vi "PulseCreateDDSSeq.vi"(8 "DDS cluster IN":T2={"DDS A Cluster"={"Seq DDS freq and phase cluster"={"Seq DDS A freq cluster"={"Ch1 start /kHz"=111053.7, "Ch1 step /kHz"=0.0, "Ch2 start /kHz"=88965.3, "Ch2 step /kHz"=0.0, "Ch3 start /kHz"=113819.6, "Ch3 step /kHz"=0.0, "Ch4 start /kHz"=86210.6, "Ch4 step /kHz"=0.0}, "Seq DDS A phase cluster"={"Ch1 phase"=0.0, "Ch1 step"=0.0, "Ch2 phase"=0.0, "Ch2"=0.0, "Ch3 phase"=0.0, "Ch3 step"=0.0, "Ch4 phase"=0.0, "Ch4 step"=0.0}}, "DDS Cluster"={"freq cluster"={"C1 freq"=110584.0, "C2 freq"=111432.0, "C3 freq"=100028.0, "C4 freq"=100021.0}, "amp cluster"={"C1 amp"=0.7, "C2 amp"=0.04, "C3 amp"=0.023, "C4 amp"=0.023}, "phase cluster"={"C1 phase"=0.0, "C2 phase"=0.0, "C3 phase"=0.0, "C4 phase"=0.0}}, "Status: "=FALSE}, "DDS B Cluster"={"Seq DDS freq and phase cluster"={"Seq DDS A freq cluster"={"Ch1 start /kHz"=111053.7, "Ch1 step /kHz"=0.0, "Ch2 start /kHz"=88965.3, "Ch2 step /kHz"=0.0, "Ch3 start /kHz"=113819.6, "Ch3 step /kHz"=0.0, "Ch4 start /kHz"=86210.6, "Ch4 step /kHz"=0.0}, "Seq DDS A phase cluster"={"Ch1 phase"=0.0, "Ch1 step"=0.0, "Ch2 phase"=0.0, "Ch2"=0.0, "Ch3 phase"=0.0, "Ch3 step"=0.0, "Ch4 phase"=0.0, "Ch4 step"=0.0}}, "DDS Cluster"={"freq cluster"={"C1 freq"=110584.0, "C2 freq"=111432.0, "C3 freq"=100028.0, "C4 freq"=100021.0}, "amp cluster"={"C1 amp"=0.7, "C2 amp"=0.04, "C3 amp"=0.023, "C4 amp"=0.023}, "phase cluster"={"C1 phase"=0.0, "C2 phase"=0.0, "C3 phase"=0.0, "C4 phase"=0.0}}, "Status: "=FALSE}, "DDS C Cluster"={"Seq DDS freq and phase cluster"={"Seq DDS A freq cluster"={"Ch1 start /kHz"=111053.7, "Ch1 step /kHz"=0.0, "Ch2 start /kHz"=88965.3, "Ch2 step /kHz"=0.0, "Ch3 start /kHz"=113819.6, "Ch3 step /kHz"=0.0, "Ch4 start /kHz"=86210.6, "Ch4 step /kHz"=0.0}, "Seq DDS A phase cluster"={"Ch1 phase"=0.0, "Ch1 step"=0.0, "Ch2 phase"=0.0, "Ch2"=0.0, "Ch3 phase"=0.0, "Ch3 step"=0.0, "Ch4 phase"=0.0, "Ch4 step"=0.0}}, "DDS Cluster"={"freq cluster"={"C1 freq"=110584.0, "C2 freq"=111432.0, "C3 freq"=100028.0, "C4 freq"=100021.0}, "amp cluster"={"C1 amp"=0.7, "C2 amp"=0.04, "C3 amp"=0.023, "C4 amp"=0.023}, "phase cluster"={"C1 phase"=0.0, "C2 phase"=0.0, "C3 phase"=0.0, "C4 phase"=0.0}}, "Status: "=FALSE}, "DDS D Cluster"={"Seq DDS freq and phase cluster"={"Seq DDS A freq cluster"={"Ch1 start /kHz"=111053.7, "Ch1 step /kHz"=0.0, "Ch2 start /kHz"=88965.3, "Ch2 step /kHz"=0.0, "Ch3 start /kHz"=113819.6, "Ch3 step /kHz"=0.0, "Ch4 start /kHz"=86210.6, "Ch4 step /kHz"=0.0}, "Seq DDS A phase cluster"={"Ch1 phase"=0.0, "Ch1 step"=0.0, "Ch2 phase"=0.0, "Ch2"=0.0, "Ch3 phase"=0.0, "Ch3 step"=0.0, "Ch4 phase"=0.0, "Ch4 step"=0.0}}, "DDS Cluster"={"freq cluster"={"C1 freq"=110584.0, "C2 freq"=111432.0, "C3 freq"=100028.0, "C4 freq"=100021.0}, "amp cluster"={"C1 amp"=0.7, "C2 amp"=0.04, "C3 amp"=0.023, "C4 amp"=0.023}, "phase cluster"={"C1 phase"=0.0, "C2 phase"=0.0, "C3 phase"=0.0, "C4 phase"=0.0}}, "Status: "=FALSE}} {"DDS D Cluster"."DDS Cluster"."phase cluster"."C4 phase" min=0.0 max=0.5; "DDS D Cluster"."DDS Cluster"."phase cluster"."C3 phase" min=0.0 max=0.5; "DDS D Cluster"."DDS Cluster"."phase cluster"."C2 phase" min=0.0 max=0.5; "DDS D Cluster"."DDS Cluster"."phase cluster"."C1 phase" min=0.0 max=0.5; "DDS D Cluster"."DDS Cluster"."amp cluster"."C4 amp" min=0.0 max=0.5; "DDS D Cluster"."DDS Cluster"."amp cluster"."C3 amp" min=0.0 max=0.5; "DDS D Cluster"."DDS Cluster"."amp cluster"."C2 amp" min=0.0 max=0.5; "DDS D Cluster"."DDS Cluster"."amp cluster"."C1 amp" min=0.0 max=0.5; "DDS D Cluster"."Seq DDS freq and phase cluster"."Seq DDS A phase cluster"."Ch4 phase" format="%#_8g"; "DDS D Cluster"."Seq DDS freq and phase cluster"."Seq DDS A phase cluster"."Ch3 phase" format="%#_8g"; "DDS D Cluster"."Seq DDS freq and phase cluster"."Seq DDS A phase cluster"."Ch2 phase" format="%#_8g"; "DDS D Cluster"."Seq DDS freq and phase cluster"."Seq DDS A phase cluster"."Ch1 phase" format="%#_8g"; "DDS D Cluster"."Seq DDS freq and phase cluster"."Seq DDS A freq cluster"."Ch4 start /kHz" format="%#_8g"; "DDS D Cluster"."Seq DDS freq and phase cluster"."Seq DDS A freq cluster"."Ch3 start /kHz" format="%#_8g"; "DDS D Cluster"."Seq DDS freq and phase cluster"."Seq DDS A freq cluster"."Ch2 start /kHz" format="%#_8g"; "DDS D Cluster"."Seq DDS freq and phase cluster"."Seq DDS A freq cluster"."Ch1 start /kHz" format="%#_8g"; "DDS C Cluster"."DDS Cluster"."phase cluster"."C4 phase" min=0.0 max=0.5; "DDS C Cluster"."DDS Cluster"."phase cluster"."C3 phase" min=0.0 max=0.5; "DDS C Cluster"."DDS Cluster"."phase cluster"."C2 phase" min=0.0 max=0.5; "DDS C Cluster"."DDS Cluster"."phase cluster"."C1 phase" min=0.0 max=0.5; "DDS C Cluster"."DDS Cluster"."amp cluster"."C4 amp" min=0.0 max=0.5; "DDS C Cluster"."DDS Cluster"."amp cluster"."C3 amp" min=0.0 max=0.5; "DDS C Cluster"."DDS Cluster"."amp cluster"."C2 amp" min=0.0 max=0.5; "DDS C Cluster"."DDS Cluster"."amp cluster"."C1 amp" min=0.0 max=0.5; "DDS C Cluster"."Seq DDS freq and phase cluster"."Seq DDS A phase cluster"."Ch4 phase" format="%#_8g"; "DDS C Cluster"."Seq DDS freq and phase cluster"."Seq DDS A phase cluster"."Ch3 phase" format="%#_8g"; "DDS C Cluster"."Seq DDS freq and phase cluster"."Seq DDS A phase cluster"."Ch2 phase" format="%#_8g"; "DDS C Cluster"."Seq DDS freq and phase cluster"."Seq DDS A phase cluster"."Ch1 phase" format="%#_8g"; "DDS C Cluster"."Seq DDS freq and phase cluster"."Seq DDS A freq cluster"."Ch4 start /kHz" format="%#_8g"; "DDS C Cluster"."Seq DDS freq and phase cluster"."Seq DDS A freq cluster"."Ch3 start /kHz" format="%#_8g"; "DDS C Cluster"."Seq DDS freq and phase cluster"."Seq DDS A freq cluster"."Ch2 start /kHz" format="%#_8g"; "DDS C Cluster"."Seq DDS freq and phase cluster"."Seq DDS A freq cluster"."Ch1 start /kHz" format="%#_8g"; "DDS B Cluster"."DDS Cluster"."phase cluster"."C4 phase" min=0.0 max=0.5; "DDS B Cluster"."DDS Cluster"."phase cluster"."C3 phase" min=0.0 max=0.5; "DDS B Cluster"."DDS Cluster"."phase cluster"."C2 phase" min=0.0 max=0.5; "DDS B Cluster"."DDS Cluster"."phase cluster"."C1 phase" min=0.0 max=0.5; "DDS B Cluster"."DDS Cluster"."amp cluster"."C4 amp" min=0.0 max=0.5; "DDS B Cluster"."DDS Cluster"."amp cluster"."C3 amp" min=0.0 max=0.5; "DDS B Cluster"."DDS Cluster"."amp cluster"."C2 amp" min=0.0 max=0.5; "DDS B Cluster"."DDS Cluster"."amp cluster"."C1 amp" min=0.0 max=0.5; "DDS B Cluster"."Seq DDS freq and phase cluster"."Seq DDS A phase cluster"."Ch4 phase" format="%#_8g"; "DDS B Cluster"."Seq DDS freq and phase cluster"."Seq DDS A phase cluster"."Ch3 phase" format="%#_8g"; "DDS B Cluster"."Seq DDS freq and phase cluster"."Seq DDS A phase cluster"."Ch2 phase" format="%#_8g"; "DDS B Cluster"."Seq DDS freq and phase cluster"."Seq DDS A phase cluster"."Ch1 phase" format="%#_8g"; "DDS B Cluster"."Seq DDS freq and phase cluster"."Seq DDS A freq cluster"."Ch4 start /kHz" format="%#_8g"; "DDS B Cluster"."Seq DDS freq and phase cluster"."Seq DDS A freq cluster"."Ch3 start /kHz" format="%#_8g"; "DDS B Cluster"."Seq DDS freq and phase cluster"."Seq DDS A freq cluster"."Ch2 start /kHz" format="%#_8g"; "DDS B Cluster"."Seq DDS freq and phase cluster"."Seq DDS A freq cluster"."Ch1 start /kHz" format="%#_8g"; "DDS A Cluster"."DDS Cluster"."phase cluster"."C4 phase" min=0.0 max=0.5; "DDS A Cluster"."DDS Cluster"."phase cluster"."C3 phase" min=0.0 max=0.5; "DDS A Cluster"."DDS Cluster"."phase cluster"."C2 phase" min=0.0 max=0.5; "DDS A Cluster"."DDS Cluster"."phase cluster"."C1 phase" min=0.0 max=0.5; "DDS A Cluster"."DDS Cluster"."amp cluster"."C4 amp" min=0.0 max=0.5; "DDS A Cluster"."DDS Cluster"."amp cluster"."C3 amp" min=0.0 max=0.5; "DDS A Cluster"."DDS Cluster"."amp cluster"."C2 amp" min=0.0 max=0.5; "DDS A Cluster"."DDS Cluster"."amp cluster"."C1 amp" min=0.0 max=0.5; "DDS A Cluster"."Seq DDS freq and phase cluster"."Seq DDS A phase cluster"."Ch4 phase" format="%#_8g"; "DDS A Cluster"."Seq DDS freq and phase cluster"."Seq DDS A phase cluster"."Ch3 phase" format="%#_8g"; "DDS A Cluster"."Seq DDS freq and phase cluster"."Seq DDS A phase cluster"."Ch2 phase" format="%#_8g"; "DDS A Cluster"."Seq DDS freq and phase cluster"."Seq DDS A phase cluster"."Ch1 phase" format="%#_8g"; "DDS A Cluster"."Seq DDS freq and phase cluster"."Seq DDS A freq cluster"."Ch4 start /kHz" format="%#_8g"; "DDS A Cluster"."Seq DDS freq and phase cluster"."Seq DDS A freq cluster"."Ch3 start /kHz" format="%#_8g"; "DDS A Cluster"."Seq DDS freq and phase cluster"."Seq DDS A freq cluster"."Ch2 start /kHz" format="%#_8g"; "DDS A Cluster"."Seq DDS freq and phase cluster"."Seq DDS A freq cluster"."Ch1 start /kHz" format="%#_8g"}) -> (0 "dds seq out":T1)   [LabVIEW 2017]
uses:
  controls/DDScontrol.ctl
  SequenceCluster.ctl
panel:
  # "DDS A"
  # "DDS B"
  # "DDS D"
  # "DDS C"
  # "MW1"
  # "MW2"
  # "MW3"
  # "MW4"
  # "Frequency [kHz]"
  # "Amplitude [0-1]"
  # "Phase"
  # "Frequency [kHz]"
  # "Freq step [kHz]"
  # "Phase"
  # "Phase step"
  # "MW1"
  # "MW2"
  # "MW3"
  # "MW4"
  # "Frequency [kHz]"
  # "Amplitude [0-1]"
  # "Phase"
  # "Frequency [kHz]"
  # "Freq step [kHz]"
  # "Phase"
  # "Phase step"
  # "MW1"
  # "MW2"
  # "MW3"
  # "MW4"
  # "Frequency [kHz]"
  # "Amplitude [0-1]"
  # "Phase"
  # "Frequency [kHz]"
  # "Freq step [kHz]"
  # "Phase"
  # "Phase step"
  # "MW1"
  # "MW2"
  # "MW3"
  # "MW4"
  # "Frequency [kHz]"
  # "Amplitude [0-1]"
  # "Phase"
  # "Frequency [kHz]"
  # "Freq step [kHz]"
  # "Phase"
  # "Phase step"
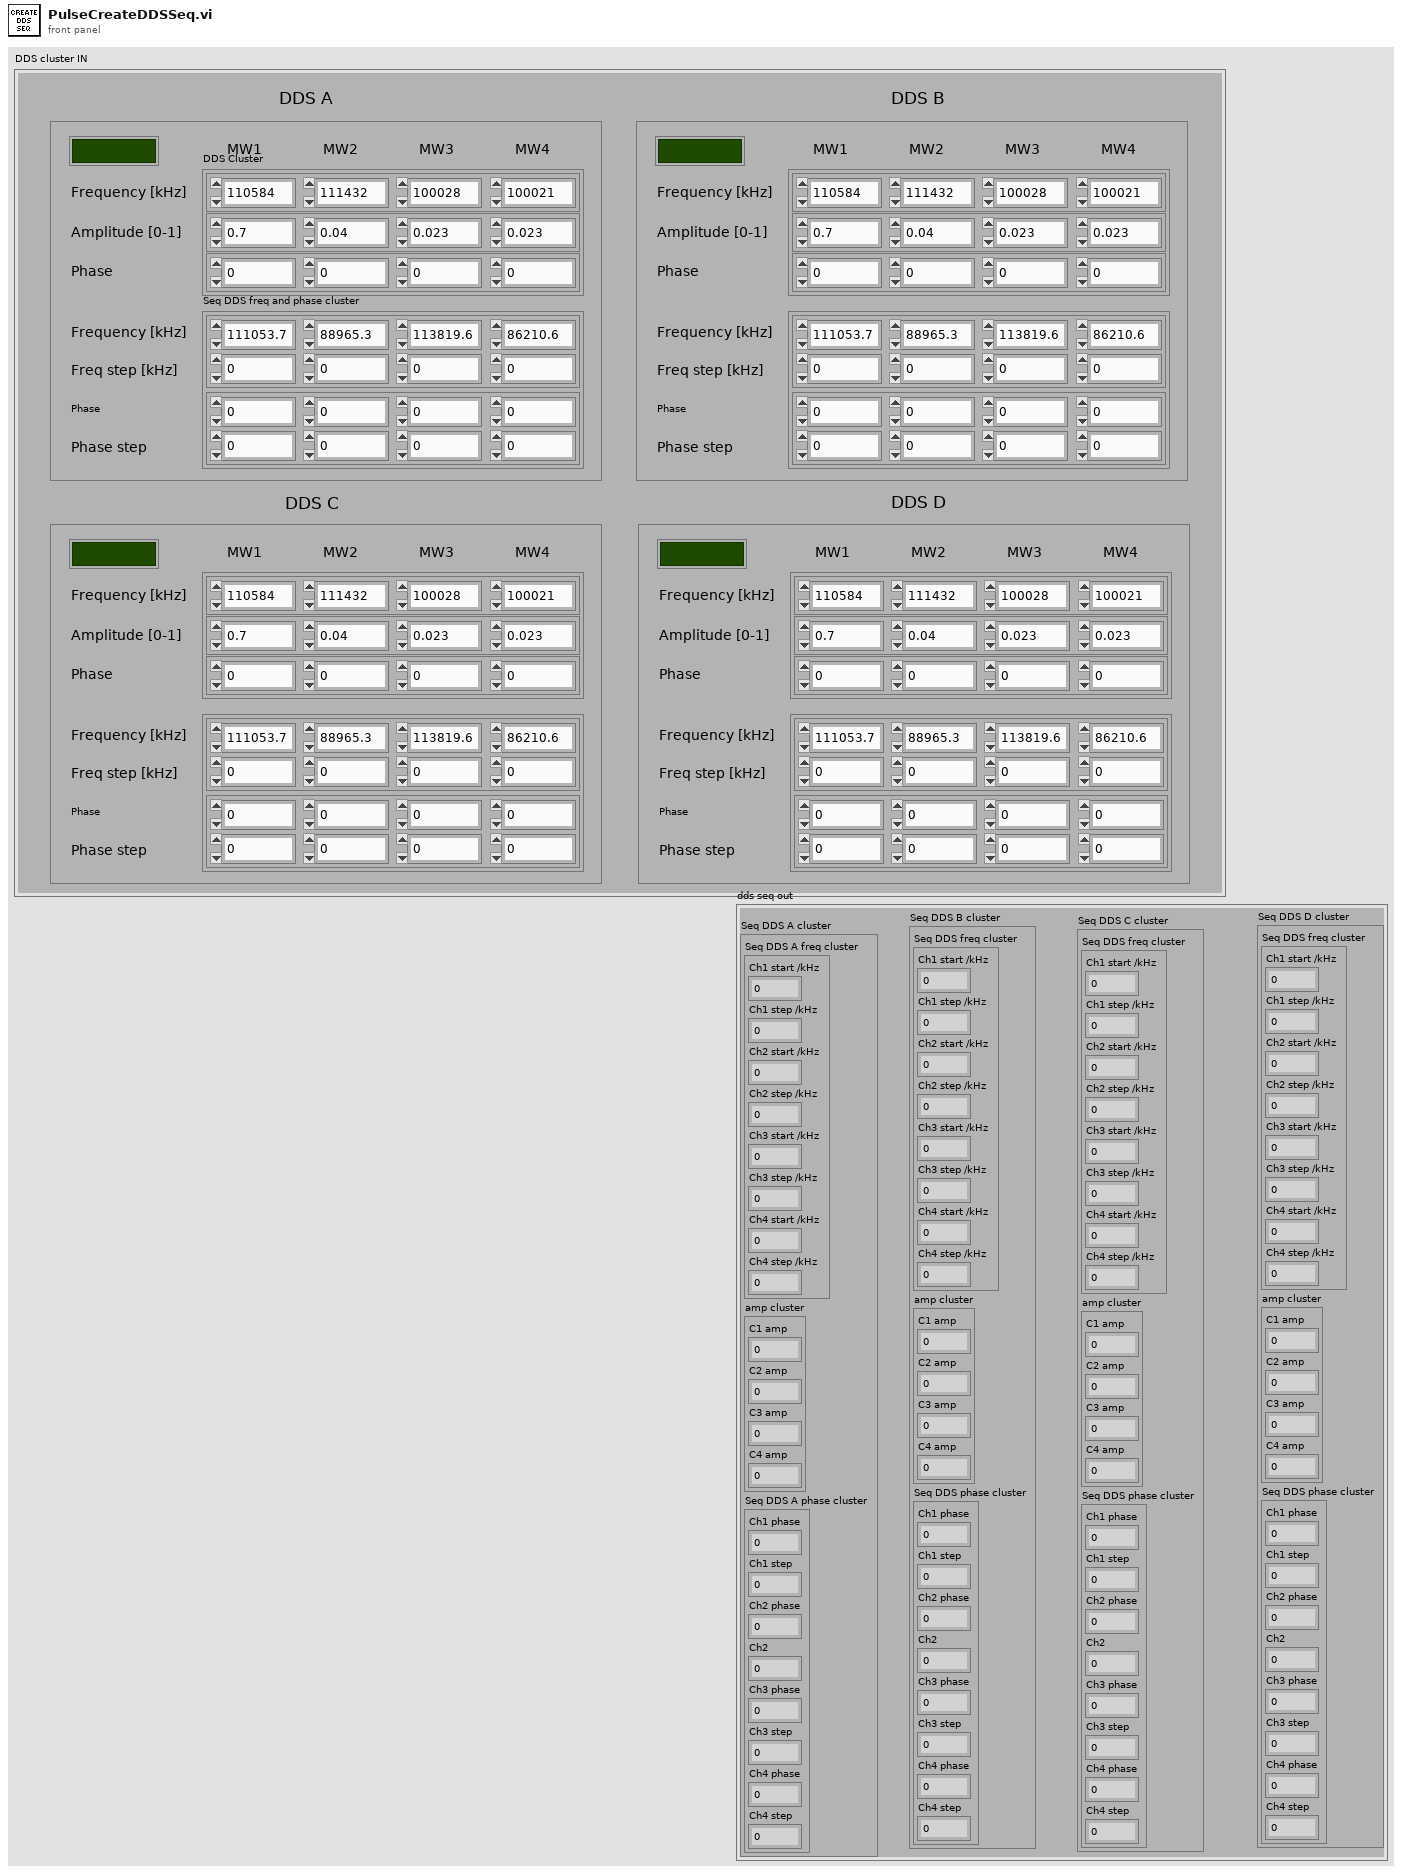
[diagram p1: front panel]
types:
  T1 = typedef "SequenceCluster.ctl" = cluster{"Seq DDS A cluster":cluster{"Seq DDS A freq cluster":cluster{"Ch1 start /kHz":dbl, "Ch1 step /kHz":dbl, "Ch2 start /kHz":dbl, "Ch2 step /kHz":dbl, "Ch3 start /kHz":dbl, "Ch3 step /kHz":dbl, "Ch4 start /kHz":dbl, "Ch4 step /kHz":dbl}, "amp cluster":cluster{"C1 amp":dbl, "C2 amp":dbl, "C3 amp":dbl, "C4 amp":dbl}, "Seq DDS A phase cluster":cluster{"Ch1 phase":dbl, "Ch1 step":dbl, "Ch2 phase":dbl, "Ch2":dbl, "Ch3 phase":dbl, "Ch3 step":dbl, "Ch4 phase":dbl, "Ch4 step":dbl}}, "Seq DDS B cluster":cluster{"Seq DDS freq cluster":cluster{"Ch1 start /kHz":dbl, "Ch1 step /kHz":dbl, "Ch2 start /kHz":dbl, "Ch2 step /kHz":dbl, "Ch3 start /kHz":dbl, "Ch3 step /kHz":dbl, "Ch4 start /kHz":dbl, "Ch4 step /kHz":dbl}, "amp cluster":cluster{"C1 amp":dbl, "C2 amp":dbl, "C3 amp":dbl, "C4 amp":dbl}, "Seq DDS phase cluster":cluster{"Ch1 phase":dbl, "Ch1 step":dbl, "Ch2 phase":dbl, "Ch2":dbl, "Ch3 phase":dbl, "Ch3 step":dbl, "Ch4 phase":dbl, "Ch4 step":dbl}}, "Seq DDS C cluster":cluster{"Seq DDS freq cluster":cluster{"Ch1 start /kHz":dbl, "Ch1 step /kHz":dbl, "Ch2 start /kHz":dbl, "Ch2 step /kHz":dbl, "Ch3 start /kHz":dbl, "Ch3 step /kHz":dbl, "Ch4 start /kHz":dbl, "Ch4 step /kHz":dbl}, "amp cluster":cluster{"C1 amp":dbl, "C2 amp":dbl, "C3 amp":dbl, "C4 amp":dbl}, "Seq DDS phase cluster":cluster{"Ch1 phase":dbl, "Ch1 step":dbl, "Ch2 phase":dbl, "Ch2":dbl, "Ch3 phase":dbl, "Ch3 step":dbl, "Ch4 phase":dbl, "Ch4 step":dbl}}, "Seq DDS D cluster":cluster{"Seq DDS freq cluster":cluster{"Ch1 start /kHz":dbl, "Ch1 step /kHz":dbl, "Ch2 start /kHz":dbl, "Ch2 step /kHz":dbl, "Ch3 start /kHz":dbl, "Ch3 step /kHz":dbl, "Ch4 start /kHz":dbl, "Ch4 step /kHz":dbl}, "amp cluster":cluster{"C1 amp":dbl, "C2 amp":dbl, "C3 amp":dbl, "C4 amp":dbl}, "Seq DDS phase cluster":cluster{"Ch1 phase":dbl, "Ch1 step":dbl, "Ch2 phase":dbl, "Ch2":dbl, "Ch3 phase":dbl, "Ch3 step":dbl, "Ch4 phase":dbl, "Ch4 step":dbl}}}
  T2 = typedef "DDScontrol.ctl" = cluster{"DDS A Cluster":cluster{"Seq DDS freq and phase cluster":cluster{"Seq DDS A freq cluster":cluster{"Ch1 start /kHz":dbl, "Ch1 step /kHz":dbl, "Ch2 start /kHz":dbl, "Ch2 step /kHz":dbl, "Ch3 start /kHz":dbl, "Ch3 step /kHz":dbl, "Ch4 start /kHz":dbl, "Ch4 step /kHz":dbl}, "Seq DDS A phase cluster":cluster{"Ch1 phase":dbl, "Ch1 step":dbl, "Ch2 phase":dbl, "Ch2":dbl, "Ch3 phase":dbl, "Ch3 step":dbl, "Ch4 phase":dbl, "Ch4 step":dbl}}, "DDS Cluster":cluster{"freq cluster":cluster{"C1 freq":dbl, "C2 freq":dbl, "C3 freq":dbl, "C4 freq":dbl}, "amp cluster":cluster{"C1 amp":dbl, "C2 amp":dbl, "C3 amp":dbl, "C4 amp":dbl}, "phase cluster":cluster{"C1 phase":dbl, "C2 phase":dbl, "C3 phase":dbl, "C4 phase":dbl}}, "Status: ":bool}, "DDS B Cluster":cluster{"Seq DDS freq and phase cluster":cluster{"Seq DDS A freq cluster":cluster{"Ch1 start /kHz":dbl, "Ch1 step /kHz":dbl, "Ch2 start /kHz":dbl, "Ch2 step /kHz":dbl, "Ch3 start /kHz":dbl, "Ch3 step /kHz":dbl, "Ch4 start /kHz":dbl, "Ch4 step /kHz":dbl}, "Seq DDS A phase cluster":cluster{"Ch1 phase":dbl, "Ch1 step":dbl, "Ch2 phase":dbl, "Ch2":dbl, "Ch3 phase":dbl, "Ch3 step":dbl, "Ch4 phase":dbl, "Ch4 step":dbl}}, "DDS Cluster":cluster{"freq cluster":cluster{"C1 freq":dbl, "C2 freq":dbl, "C3 freq":dbl, "C4 freq":dbl}, "amp cluster":cluster{"C1 amp":dbl, "C2 amp":dbl, "C3 amp":dbl, "C4 amp":dbl}, "phase cluster":cluster{"C1 phase":dbl, "C2 phase":dbl, "C3 phase":dbl, "C4 phase":dbl}}, "Status: ":bool}, "DDS C Cluster":cluster{"Seq DDS freq and phase cluster":cluster{"Seq DDS A freq cluster":cluster{"Ch1 start /kHz":dbl, "Ch1 step /kHz":dbl, "Ch2 start /kHz":dbl, "Ch2 step /kHz":dbl, "Ch3 start /kHz":dbl, "Ch3 step /kHz":dbl, "Ch4 start /kHz":dbl, "Ch4 step /kHz":dbl}, "Seq DDS A phase cluster":cluster{"Ch1 phase":dbl, "Ch1 step":dbl, "Ch2 phase":dbl, "Ch2":dbl, "Ch3 phase":dbl, "Ch3 step":dbl, "Ch4 phase":dbl, "Ch4 step":dbl}}, "DDS Cluster":cluster{"freq cluster":cluster{"C1 freq":dbl, "C2 freq":dbl, "C3 freq":dbl, "C4 freq":dbl}, "amp cluster":cluster{"C1 amp":dbl, "C2 amp":dbl, "C3 amp":dbl, "C4 amp":dbl}, "phase cluster":cluster{"C1 phase":dbl, "C2 phase":dbl, "C3 phase":dbl, "C4 phase":dbl}}, "Status: ":bool}, "DDS D Cluster":cluster{"Seq DDS freq and phase cluster":cluster{"Seq DDS A freq cluster":cluster{"Ch1 start /kHz":dbl, "Ch1 step /kHz":dbl, "Ch2 start /kHz":dbl, "Ch2 step /kHz":dbl, "Ch3 start /kHz":dbl, "Ch3 step /kHz":dbl, "Ch4 start /kHz":dbl, "Ch4 step /kHz":dbl}, "Seq DDS A phase cluster":cluster{"Ch1 phase":dbl, "Ch1 step":dbl, "Ch2 phase":dbl, "Ch2":dbl, "Ch3 phase":dbl, "Ch3 step":dbl, "Ch4 phase":dbl, "Ch4 step":dbl}}, "DDS Cluster":cluster{"freq cluster":cluster{"C1 freq":dbl, "C2 freq":dbl, "C3 freq":dbl, "C4 freq":dbl}, "amp cluster":cluster{"C1 amp":dbl, "C2 amp":dbl, "C3 amp":dbl, "C4 amp":dbl}, "phase cluster":cluster{"C1 phase":dbl, "C2 phase":dbl, "C3 phase":dbl, "C4 phase":dbl}}, "Status: ":bool}}
  T3 = cluster{"Seq DDS freq and phase cluster":cluster{"Seq DDS A freq cluster":cluster{"Ch1 start /kHz":dbl, "Ch1 step /kHz":dbl, "Ch2 start /kHz":dbl, "Ch2 step /kHz":dbl, "Ch3 start /kHz":dbl, "Ch3 step /kHz":dbl, "Ch4 start /kHz":dbl, "Ch4 step /kHz":dbl}, "Seq DDS A phase cluster":cluster{"Ch1 phase":dbl, "Ch1 step":dbl, "Ch2 phase":dbl, "Ch2":dbl, "Ch3 phase":dbl, "Ch3 step":dbl, "Ch4 phase":dbl, "Ch4 step":dbl}}, "DDS Cluster":cluster{"freq cluster":cluster{"C1 freq":dbl, "C2 freq":dbl, "C3 freq":dbl, "C4 freq":dbl}, "amp cluster":cluster{"C1 amp":dbl, "C2 amp":dbl, "C3 amp":dbl, "C4 amp":dbl}, "phase cluster":cluster{"C1 phase":dbl, "C2 phase":dbl, "C3 phase":dbl, "C4 phase":dbl}}, "Status: ":bool}[]
  T4 = cluster{"Seq DDS A freq cluster":cluster{"Ch1 start /kHz":dbl, "Ch1 step /kHz":dbl, "Ch2 start /kHz":dbl, "Ch2 step /kHz":dbl, "Ch3 start /kHz":dbl, "Ch3 step /kHz":dbl, "Ch4 start /kHz":dbl, "Ch4 step /kHz":dbl}, "Seq DDS A phase cluster":cluster{"Ch1 phase":dbl, "Ch1 step":dbl, "Ch2 phase":dbl, "Ch2":dbl, "Ch3 phase":dbl, "Ch3 step":dbl, "Ch4 phase":dbl, "Ch4 step":dbl}}
  T5 = cluster{"freq cluster":cluster{"C1 freq":dbl, "C2 freq":dbl, "C3 freq":dbl, "C4 freq":dbl}, "amp cluster":cluster{"C1 amp":dbl, "C2 amp":dbl, "C3 amp":dbl, "C4 amp":dbl}, "phase cluster":cluster{"C1 phase":dbl, "C2 phase":dbl, "C3 phase":dbl, "C4 phase":dbl}}
  T6 = cluster{"Ch1 start /kHz":dbl, "Ch1 step /kHz":dbl, "Ch2 start /kHz":dbl, "Ch2 step /kHz":dbl, "Ch3 start /kHz":dbl, "Ch3 step /kHz":dbl, "Ch4 start /kHz":dbl, "Ch4 step /kHz":dbl}
  T7 = cluster{"Ch1 phase":dbl, "Ch1 step":dbl, "Ch2 phase":dbl, "Ch2":dbl, "Ch3 phase":dbl, "Ch3 step":dbl, "Ch4 phase":dbl, "Ch4 step":dbl}
  T8 = cluster{"C1 amp":dbl, "C2 amp":dbl, "C3 amp":dbl, "C4 amp":dbl}
  T9 = cluster{"Seq DDS A freq cluster":cluster{"Ch1 start /kHz":dbl, "Ch1 step /kHz":dbl, "Ch2 start /kHz":dbl, "Ch2 step /kHz":dbl, "Ch3 start /kHz":dbl, "Ch3 step /kHz":dbl, "Ch4 start /kHz":dbl, "Ch4 step /kHz":dbl}, "amp cluster":cluster{"C1 amp":dbl, "C2 amp":dbl, "C3 amp":dbl, "C4 amp":dbl}, "Seq DDS A phase cluster":cluster{"Ch1 phase":dbl, "Ch1 step":dbl, "Ch2 phase":dbl, "Ch2":dbl, "Ch3 phase":dbl, "Ch3 step":dbl, "Ch4 phase":dbl, "Ch4 step":dbl}}
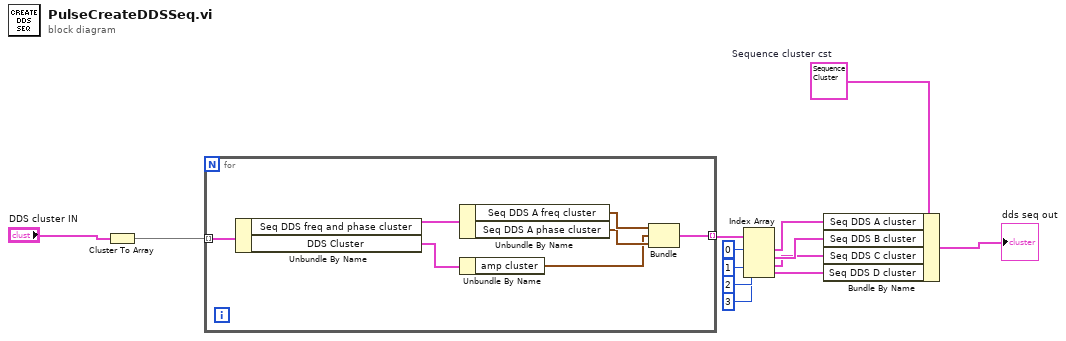
[diagram p0: block diagram]
diagram:
  w13 = T1 {"Seq DDS A cluster"={"Seq DDS A freq cluster"={"Ch1 start /kHz"=0.0, "Ch1 step /kHz"=0.0, "Ch2 start /kHz"=0.0, "Ch2 step /kHz"=0.0, "Ch3 start /kHz"=0.0, "Ch3 step /kHz"=0.0, "Ch4 start /kHz"=0.0, "Ch4 step /kHz"=0.0}, "amp cluster"={"C1 amp"=0.0, "C2 amp"=0.0, "C3 amp"=0.0, "C4 amp"=0.0}, "Seq DDS A phase cluster"={"Ch1 phase"=0.0, "Ch1 step"=0.0, "Ch2 phase"=0.0, "Ch2"=0.0, "Ch3 phase"=0.0, "Ch3 step"=0.0, "Ch4 phase"=0.0, "Ch4 step"=0.0}}, "Seq DDS B cluster"={"Seq DDS freq cluster"={"Ch1 start /kHz"=0.0, "Ch1 step /kHz"=0.0, "Ch2 start /kHz"=0.0, "Ch2 step /kHz"=0.0, "Ch3 start /kHz"=0.0, "Ch3 step /kHz"=0.0, "Ch4 start /kHz"=0.0, "Ch4 step /kHz"=0.0}, "amp cluster"={"C1 amp"=0.0, "C2 amp"=0.0, "C3 amp"=0.0, "C4 amp"=0.0}, "Seq DDS phase cluster"={"Ch1 phase"=0.0, "Ch1 step"=0.0, "Ch2 phase"=0.0, "Ch2"=0.0, "Ch3 phase"=0.0, "Ch3 step"=0.0, "Ch4 phase"=0.0, "Ch4 step"=0.0}}, "Seq DDS C cluster"={"Seq DDS freq cluster"={"Ch1 start /kHz"=0.0, "Ch1 step /kHz"=0.0, "Ch2 start /kHz"=0.0, "Ch2 step /kHz"=0.0, "Ch3 start /kHz"=0.0, "Ch3 step /kHz"=0.0, "Ch4 start /kHz"=0.0, "Ch4 step /kHz"=0.0}, "amp cluster"={"C1 amp"=0.0, "C2 amp"=0.0, "C3 amp"=0.0, "C4 amp"=0.0}, "Seq DDS phase cluster"={"Ch1 phase"=0.0, "Ch1 step"=0.0, "Ch2 phase"=0.0, "Ch2"=0.0, "Ch3 phase"=0.0, "Ch3 step"=0.0, "Ch4 phase"=0.0, "Ch4 step"=0.0}}, "Seq DDS D cluster"={"Seq DDS freq cluster"={"Ch1 start /kHz"=0.0, "Ch1 step /kHz"=0.0, "Ch2 start /kHz"=0.0, "Ch2 step /kHz"=0.0, "Ch3 start /kHz"=0.0, "Ch3 step /kHz"=0.0, "Ch4 start /kHz"=0.0, "Ch4 step /kHz"=0.0}, "amp cluster"={"C1 amp"=0.0, "C2 amp"=0.0, "C3 amp"=0.0, "C4 amp"=0.0}, "Seq DDS phase cluster"={"Ch1 phase"=0.0, "Ch1 step"=0.0, "Ch2 phase"=0.0, "Ch2"=0.0, "Ch3 phase"=0.0, "Ch3 step"=0.0, "Ch4 phase"=0.0, "Ch4 step"=0.0}}}  # Sequence cluster cst
  n1 = Cluster To Array(cluster="DDS cluster IN") -> (array=w11:T3)
  n2 = for {
    tunnel: w11 -> [w18] mode=indexing
    tunnel: [w14] -> w10 mode=indexing
    n3 = Unbundle By Name(w18) -> ("Seq DDS freq and phase cluster"=w20:T4, "DDS Cluster"=w19:T5)
    n4 = Unbundle By Name(w20) -> ("Seq DDS A freq cluster"=w17:T6, "Seq DDS A phase cluster"=w16:T7)
    n5 = Unbundle By Name(w19) -> ("amp cluster"=w15:T8)
    n6 = Bundle("Seq DDS A freq cluster"=w17, "amp cluster"=w15, "Seq DDS A phase cluster"=w16) -> (w14:T9)  [unwired: 1 in]
  }
  n7 = Index Array(array=w10, index #1=0 ("index"), index #2=1 ("index"), index #3=2 ("index"), index #4=3 ("index")) -> (element #1=w9:T9, element #2=w8:T9, element #3=w7:T9, element #4=w6:T9)
  n8 = Bundle By Name(cluster=w13, "Seq DDS A cluster"=w9, "Seq DDS B cluster"=w8, "Seq DDS C cluster"=w7, "Seq DDS D cluster"=w6) -> (→"dds seq out":T1)
